vi "ex3_producer_consumer.vi"() -> ()   [LabVIEW 2022 SP3]
uses:
  pylabview/pythonq.lvlib
  C:/Program Files (x86)/National Instruments/LabVIEW 2022/examples/Connectivity/Python/support/PythonVersionsEnum.ctl
  py_msg.ctl
panel:
  out "cur ref 2":string
  out "error out 2":errorcluster
  out "Wv 2":dbl(graph)
  out "cur ref":string
  out "count 1":i32
  in  "wait":u32=500
  out "Wv":dbl(graph)
  in  "stop":bool
  out "count 2":i32
  out "error out":errorcluster
  # "# Created by Jeff Morgan\n# https://awakeniot.com/"
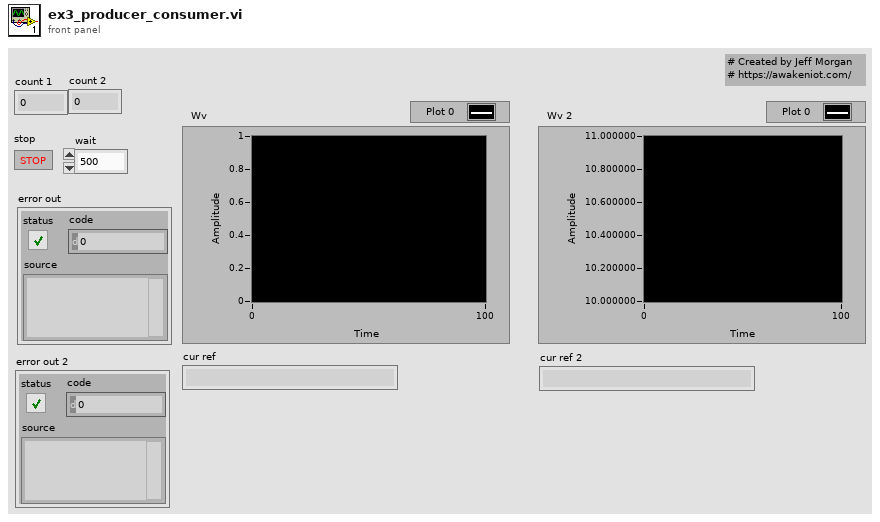
[diagram p1: front panel]
types:
  T1 = typedef "PythonVersionsEnum.ctl" = enum16{"3.6", "3.7", "3.8", "3.9"}
  T2 = typedef "pythonq.lvlib/py_cluster.ctl" = cluster{"path":path, "py":T3}
  T3 = typedef "pythonq.lvlib/py_session.ctl" = cluster{"session":refnum<k35>, "object":refnum<k38>}
  T4 = typedef "py_msg.ctl" = cluster{"double":dbl, "ref":string}
  T5 = typedef "pythonq.lvlib/py_result.ctl" = cluster{"value":string, "ok":bool, "error_msg":string}
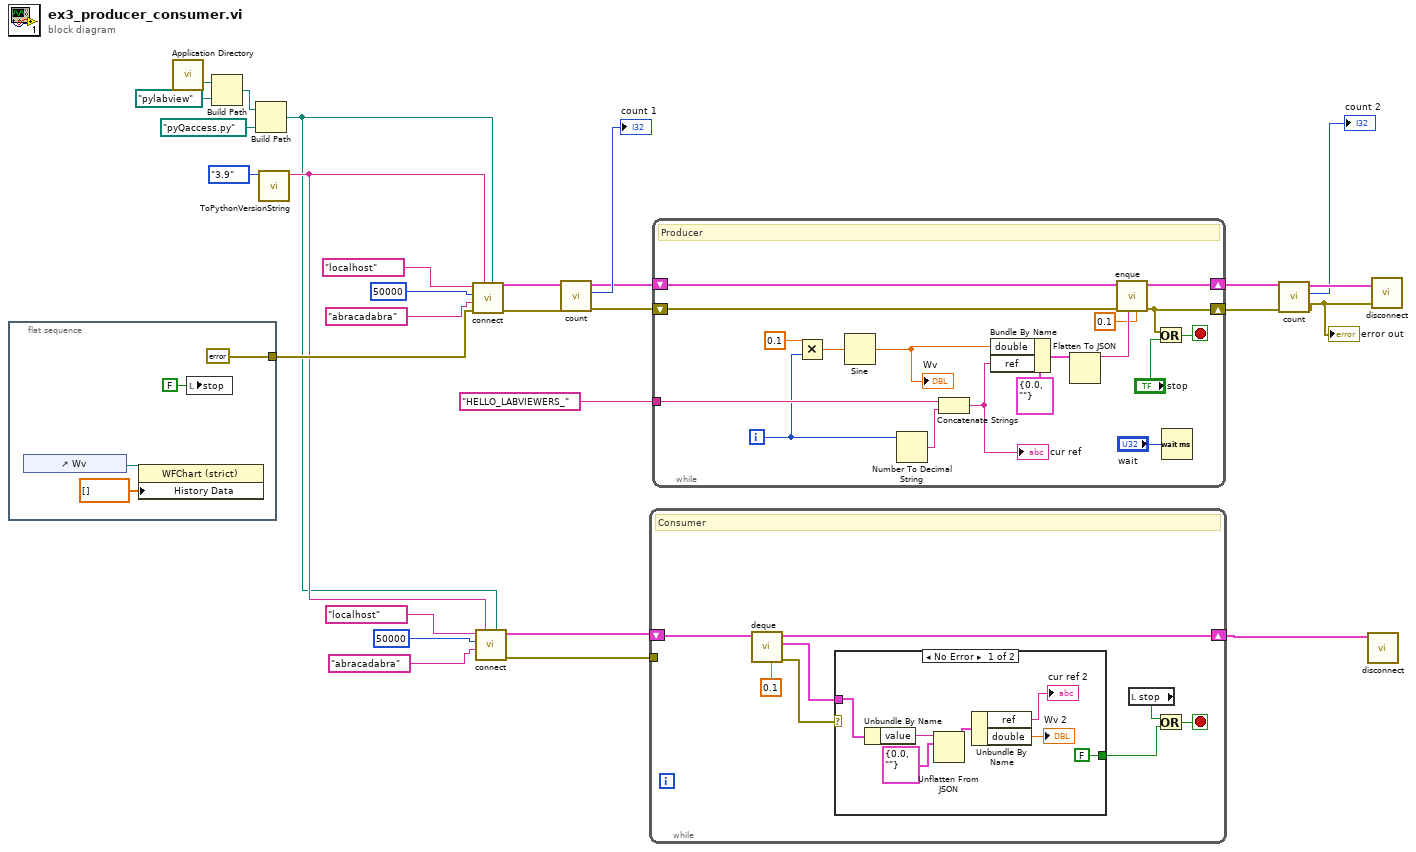
[diagram p0: block diagram]
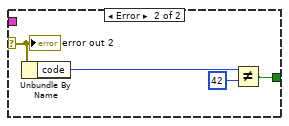
[diagram p2: hidden frame]
diagram:
  n1 = flat-sequence {
    tunnel: [errorcluster {"status"=FALSE, "code"=0, "source"=""} ("error in (no error)")] -> w15
    frame #0 {
      n2 = control-ref of="Wv"() -> (w30:refnum<vi>)
      n3 = property class="WFChart (strict)"(reference=w30, "History Data"=dbl[] []) -> ()  [unwired: 1 in, 2 out]
      n4 = local write "stop"(FALSE ("stop")) -> ()
    }
  }
  n5 = call <vilib>:"Application Directory.vi"() -> ("Application Directory"=w23:path)
  n6 = Build Path(base path=w23, name or relative path=path "pylabview") -> (appended path=w24:path)
  n7 = Build Path(base path=w24, name or relative path=path "pyQaccess.py") -> (appended path=w5:path)
  n8 = call "ToPythonVersionString.vi"("python version"=PythonVersionsEnum."3.9") -> ("python version string"=w6:string)  [unwired: 10 in]
  n9 = call "connect.vi"("module path"=w5, "Python version"=w6, "error in (no error)"=w15, "password"="abracadabra", "port"=50000, "ip_address"="localhost") -> ("error out"=w18:errorcluster, "py out"=w17:T2)  [unwired: 4 in]
  n10 = call "connect.vi"("module path"=w5, "Python version"=w6, "password"="abracadabra", "port"=50000, "ip_address"="localhost") -> ("error out"=w3:errorcluster, "py out"=w4:T2)  [unwired: 5 in]
  n11 = call "count.vi"("error in (no error)"=w18, "py in"=w17) -> ("error out"=w14:errorcluster, "count"=→"count 1":i32, "py out"=w10:T2)  [unwired: 7 in]
  n12 = while {
    shift-right: [w39] -> w1
    shift-left: w4 -> [w40]
    tunnel: w3 -> [_]
    stop <- w36 stop-if-true
    # "Consumer"
    n13 = call "deque.vi"("timeout"=0.1, "py in"=w40) -> ("error out"=w37:errorcluster, "response"=w34:T5, "py out"=w39:T2)  [unwired: 6 in, 1 out]
    n14 = case shown="No Error" w37 {
      selector: w37 -> [_ w51]
      tunnel: [FALSE w48] -> w35
      tunnel: w34 -> [w46 _]
      frame No Error {
        n15 = Unbundle By Name(w46) -> ("value"=w45:string)
        n16 = Unflatten From JSON(JSON string=w45, type and defaults=T4 {"double"=0.0, "ref"=""} ("Cluster")) -> (value=w43:T4)  [unwired: 5 in, 1 out]
        n17 = Unbundle By Name(w43) -> ("ref"=→"cur ref 2":string, "double"=→"Wv 2":dbl)
      }
      frame Error {
        n18 = Unbundle By Name(w51) -> ("code"=w50:i32)
        n19 = Not Equal?(x=w50, y=42) -> (x != y?=w48:bool)
        "error out 2" <- w51
      }
    }
    n20 = local read "stop"() -> (w33:bool)
    n21 = Or(x=w33, y=w35) -> (x .or. y?=w36:bool)
  }
  n22 = while {
    shift-right: [w68] -> w2
    shift-left: w10 -> [w69]
    shift-right: [w65] -> w16
    shift-left: w14 -> [w67]
    tunnel: "HELLO_LABVIEWERS_" ("ref_prefix") -> [w62]
    i -> [w53]
    stop <- w66 stop-if-true
    # "Producer"
    n23 = Multiply(x=0.1, y=w53) -> (x*y=w54:dbl)
    n24 = Sine(x=w54) -> (sin(x)=w52:dbl)
    "Wv" <- w52
    n25 = Number To Decimal String(number=w53) -> (decimal integer string=w61:string)  [unwired: 1 in]
    n26 = Concatenate Strings(w62, w61) -> (w59:string)
    "cur ref" <- w59
    n27 = Bundle By Name(cluster=T4 {"double"=0.0, "ref"=""} ("Cluster"), "double"=w52, "ref"=w59) -> (w58:T4)
    n28 = Flatten To JSON(anything=w58) -> (JSON string=w57:string)  [unwired: 2 in, 1 out]
    n29 = call "enque.vi"("timeout"=0.1, "data in"=w57, "error in (no error)"=w67, "py in"=w69) -> ("error out"=w65:errorcluster, "py out"=w68:T2)  [unwired: 4 in, 2 out]
    n30 = Or(x=w65, y="stop") -> (x .or. y?=w66:bool)
    n31 = Wait (ms)(milliseconds to wait="wait") -> ()  [unwired: 1 out]
  }
  n32 = call "count.vi"("error in (no error)"=w16, "py in"=w2) -> ("error out"=w12:errorcluster, "count"=→"count 2":i32, "py out"=w20:T2)  [unwired: 7 in]
  "error out" <- w12
  n33 = call "disconnect.vi"("py in"=w1) -> ()  [unwired: 10 in, 1 out]
  n34 = call "disconnect.vi"("error in (no error)"=w12, "py in"=w20) -> ()  [unwired: 9 in, 1 out]
